vi "HardwareLoop.vi"(8 "Error In":errorcluster, 9 "Executable Configuration":T2, 10 "Data Structures":T1, 11 "Action Queues":T3) -> (0 "Error Out":errorcluster)   [LabVIEW 2012]
uses:
  ActionQueues.ctl
  UIActionQueueElement.ctl
  UIAction.ctl
  HardwareActionQueueElement.ctl
  HardwareAction.ctl
  LogActionQueueElement.ctl
  LogAction.ctl
  ExecutableConfiguration.ctl
  DataStructures.ctl
  HardwareDisplayData.ctl
  HardwareLogData.ctl
  Setup.ctl
  DUTConfiguration.ctl
  driver/Public/Controls/SMUSense.ctl
  LogConfiguration.ctl
  LogStartConfiguration.ctl
  LogStartTriggerType.ctl
  LogDigitalIOTriggerEdge.ctl
  LogRolloverConfiguration.ctl
  LogRolloverTriggerType.ctl
  LogStopConfiguration.ctl
  LogStopTriggerType.ctl
  TriggerConfiguration.ctl
  TriggerInputConfiguration.ctl
  TriggerInputType.ctl
  driver/Public/Controls/TriggerMode.ctl
  TriggerOutputConfiguration.ctl
  TriggerOutputType.ctl
  SourceConfiguration.ctl
  SourceFunction.ctl
  MeasureConfiguration.ctl
  HardwareAbortGlobalAction.ctl
  <vilib>/Utility/error.llb/DialogType.ctl
  driver/Keithley-2602.lvlib
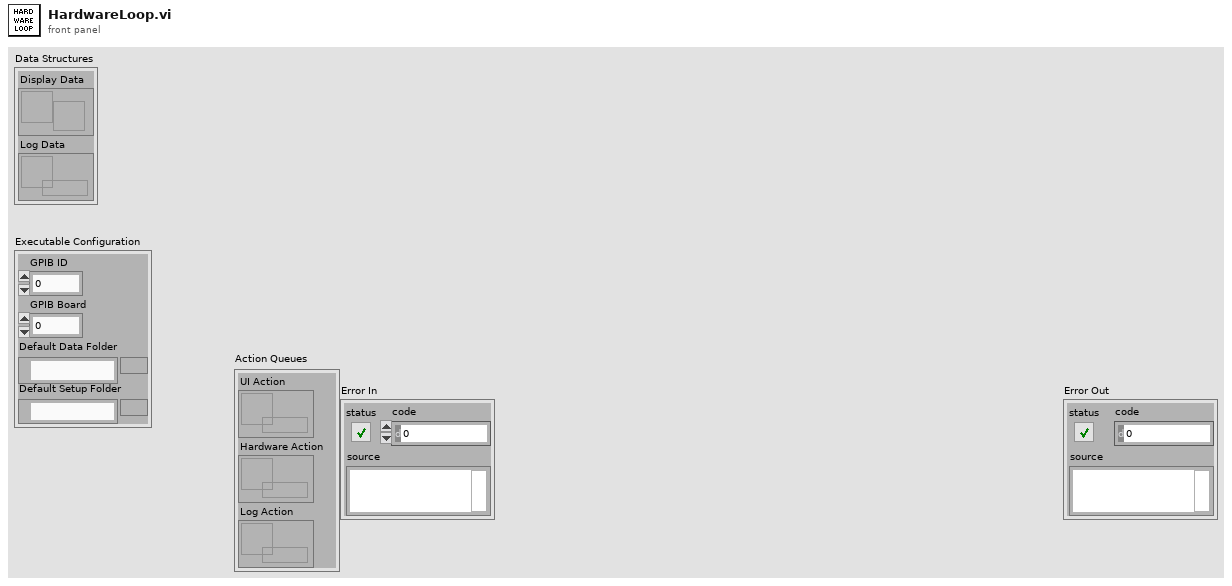
[diagram p1: front panel]
types:
  T1 = typedef "DataStructures.ctl" = cluster{"Display Data":refnum<notifier>, "Log Data":refnum<queue>}
  T2 = typedef "ExecutableConfiguration.ctl" = cluster{"GPIB ID":u8, "GPIB Board":u8, "Default Data Folder":path, "Default Setup Folder":path}
  T3 = typedef "ActionQueues.ctl" = cluster{"UI Action":refnum<queue>, "Hardware Action":refnum<queue>, "Log Action":refnum<queue>}
  T4 = typedef "Setup.ctl" = cluster{"DUT":T5, "Log":T7, "Trigger":T15, "Sources":T21[], "Measures":T23[]}
  T5 = typedef "DUTConfiguration.ctl" = cluster{"Count":u32, "Wirings":T6[], "Names":string[][]}
  T6 = typedef "Keithley-2602.lvlib/SMUSense.ctl" = enum16{"Local (2-wire)", "Remote (4-wire)", "Calibration"}
  T7 = typedef "LogConfiguration.ctl" = cluster{"Start":T8, "Rollover":T11, "Stop":T13}
  T8 = typedef "LogStartConfiguration.ctl" = cluster{"Trigger Type":T9, "Timer (sec)":dbl, "Digital IO Line":u8, "Digital IO Edge":T10}
  T9 = typedef "LogStartTriggerType.ctl" = enum16{"Immediate", "User", "Timer", "Digital IO"}
  T10 = typedef "LogDigitalIOTriggerEdge.ctl" = enum16{"Rising", "Falling"}
  T11 = typedef "LogRolloverConfiguration.ctl" = cluster{"Trigger Type":T12, "Timer (sec)":dbl, "File Size (MB)":u32, "Digital IO Line":u8, "Digital IO Edge":T10}
  T12 = typedef "LogRolloverTriggerType.ctl" = enum16{"None", "Timer", "File Size", "Digital IO"}
  T13 = typedef "LogStopConfiguration.ctl" = cluster{"Trigger Type":T14, "Timer (sec)":dbl, "File Size (MB)":u32, "Digital IO Line":u8, "Digital IO Edge":T10}
  T14 = typedef "LogStopTriggerType.ctl" = enum16{"None", "User", "Timer", "File Size", "Digital IO"}
  T15 = typedef "TriggerConfiguration.ctl" = cluster{"Input":T16, "Output":T19}
  T16 = typedef "TriggerInputConfiguration.ctl" = cluster{"Type":T17, "Timeout (ms)":u32, "Delay (ms)":u32, "Digital IO Line (1-14)":u8, "Digital IO Mode":T18}
  T17 = typedef "TriggerInputType.ctl" = enum16{"None", "Digital IO", "Bus"}
  T18 = typedef "Keithley-2602.lvlib/TriggerMode.ctl" = enum16{"Falling", "Rising", "Either", "Synchronous"}
  T19 = typedef "TriggerOutputConfiguration.ctl" = cluster{"Type":T20, "Delay (ms)":u32, "Digital IO Line (1-14)":u8, "Digital IO Mode":T18, "Digital IO Pulse Width (sec)":dbl}
  T20 = typedef "TriggerOutputType.ctl" = enum16{"None", "Digital IO", "Bus"}
  T21 = typedef "SourceConfiguration.ctl" = cluster{"Enabled?":bool, "Function":T22, "Level (V or A)":dbl, "Autorange Enabled?":bool, "High Limit (V or A)":dbl, "Low Limit (V or A)":dbl}
  T22 = typedef "SourceFunction.ctl" = enum16{"Voltage", "Current"}
  T23 = typedef "MeasureConfiguration.ctl" = cluster{"Enabled?":bool, "Count":u8, "Interval (sec)":dbl, "Voltage Auto Range Enabled?":bool, "Voltage High Limit (V or A)":dbl, "Voltage Low Limit (V or A)":dbl, "Current Auto Range Enabled?":bool, "Current High Limit (V or A)":dbl, "Current Low Limit (V or A)":dbl}
  T24 = typedef "HardwareActionQueueElement.ctl" = cluster{"Action":T25, "Data":variant}
  T25 = typedef "HardwareAction.ctl" = enum16{"Initialize", "Start", "Run", "Stop", "Error", "Shutdown"}
  T26 = typedef "UIActionQueueElement.ctl" = cluster{"Action":T27, "Data":variant}
  T27 = typedef "UIAction.ctl" = enum16{"Initialize", "Configure Trigger", "Configure Measure", "Configure Source", "Configure DUT", "Configure Log", "Configure Open", "Configure Save", "Configure Reset", "Hardware Start", "Hardware Started", "Hardware Stop", "Hardware Stopped", "Log Arm", "Log Start", "Log Started", "Log Stop", "Log Stopped", "Create Chart", "Error", "Shutdown"}
  T28 = typedef "HardwareLogData.ctl" = cluster{"Timestamp":timestamp, "Data":T29}
  T29 = typedef "HardwareDisplayData.ctl" = cluster{"DUT Names":string[][], "SMU":dbl[][], "Port":bool[]}
  T30 = typedef "HardwareAbortGlobalAction.ctl" = enum16{"Set", "Get"}
  T31 = typedef "DialogType.ctl" = u16
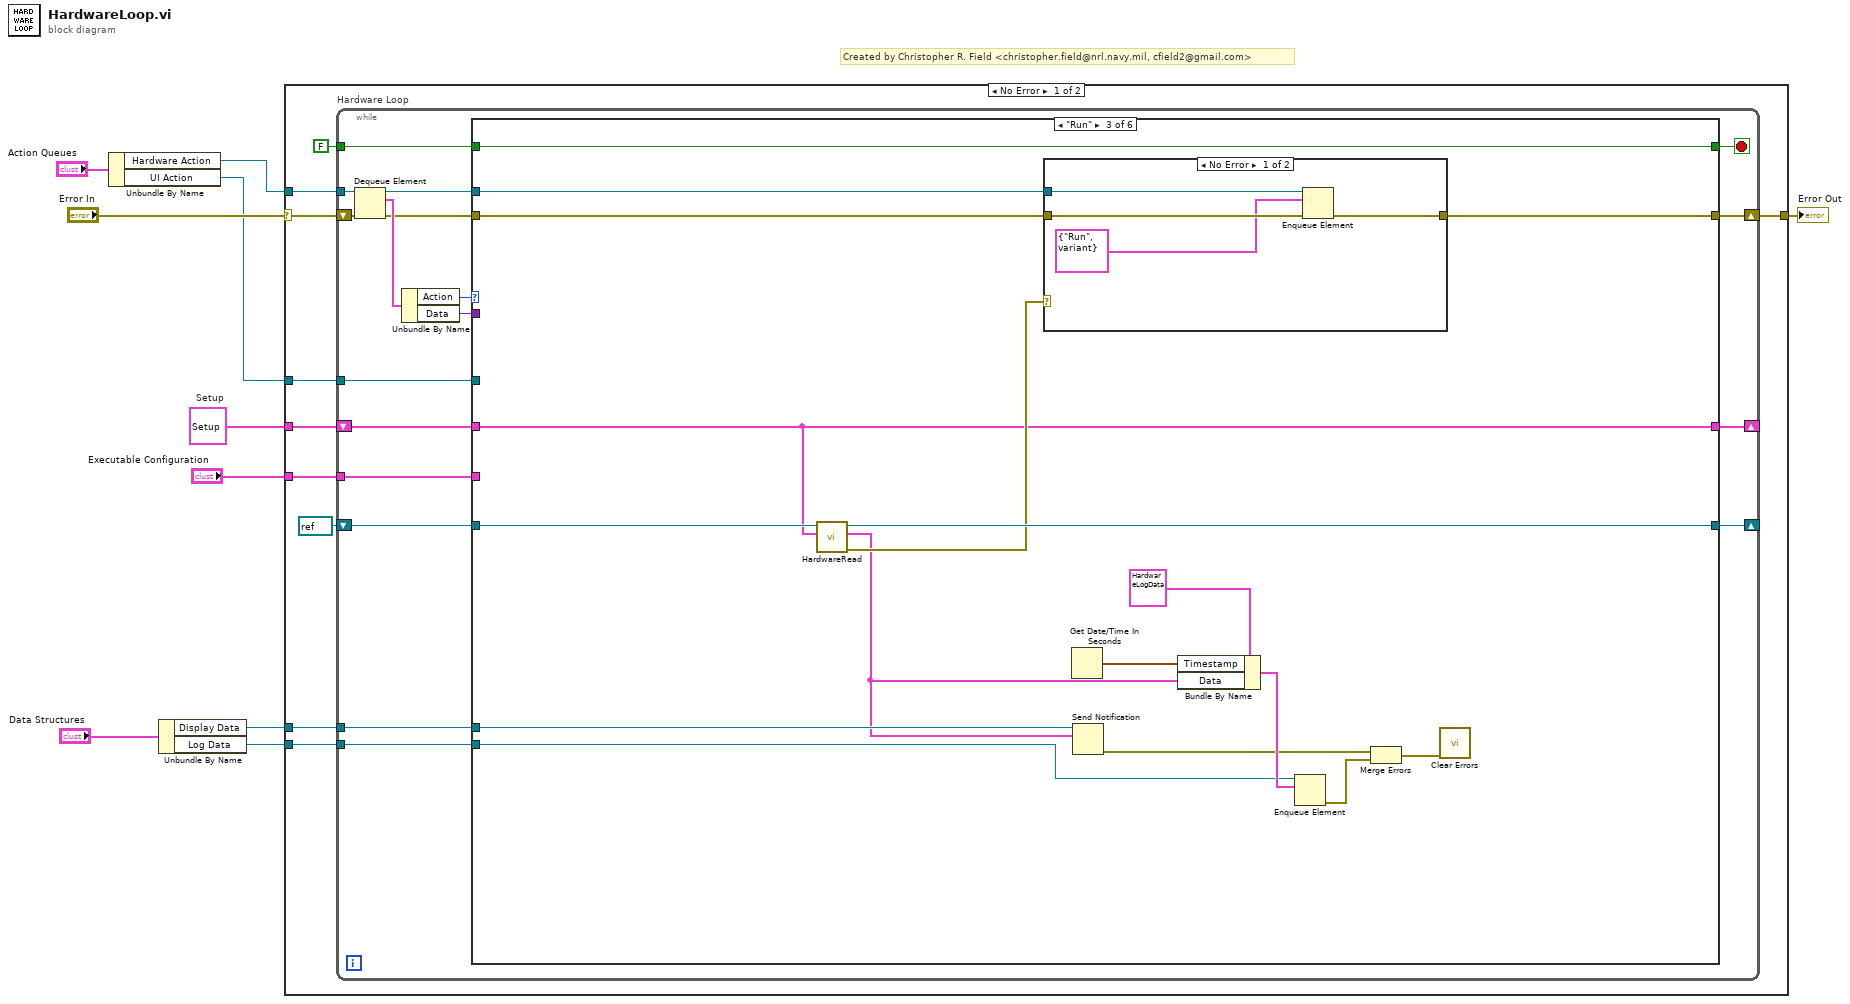
[diagram p0: block diagram]
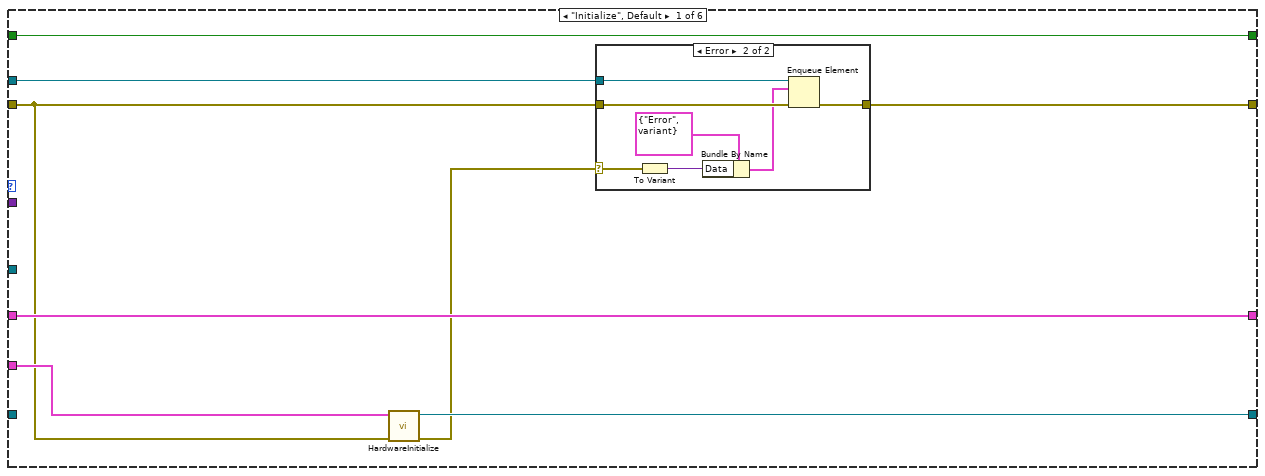
[diagram p2: hidden frame]
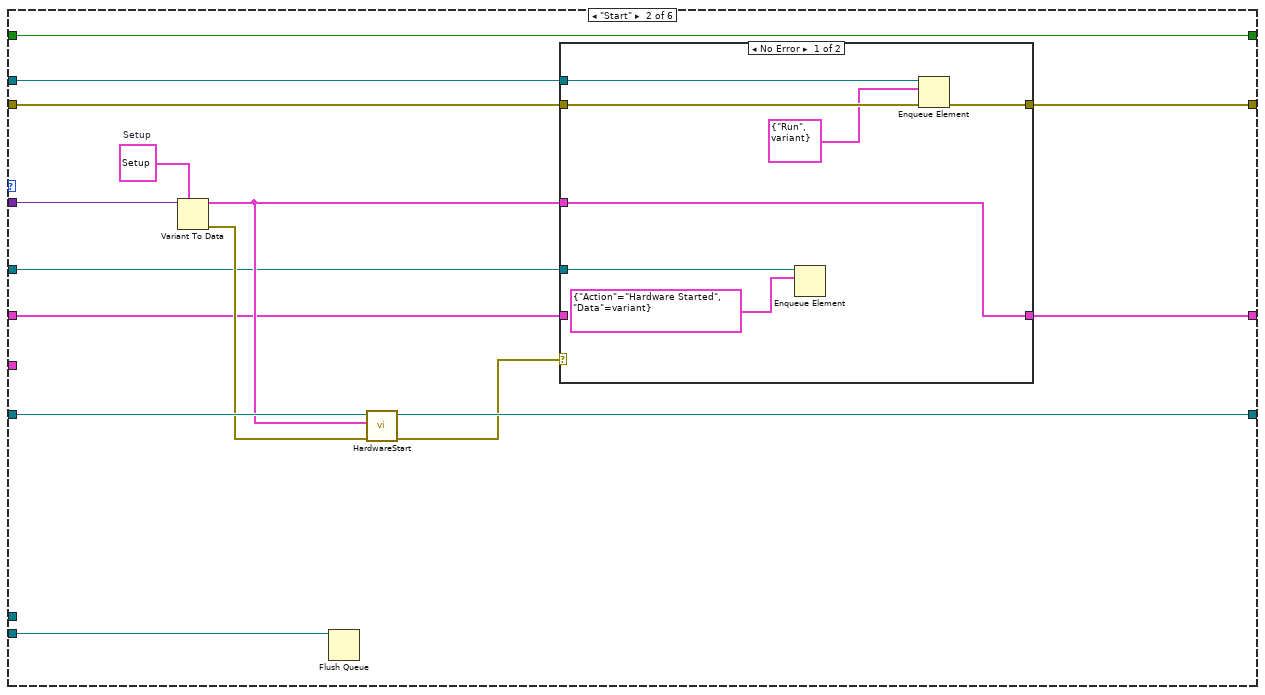
[diagram p4: hidden frame]
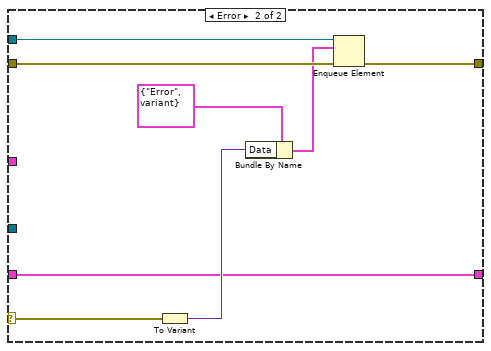
[diagram p5: hidden frame]
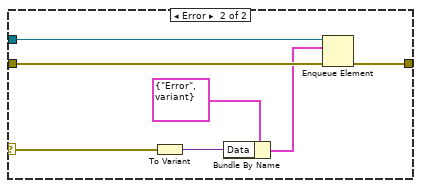
[diagram p6: hidden frame]
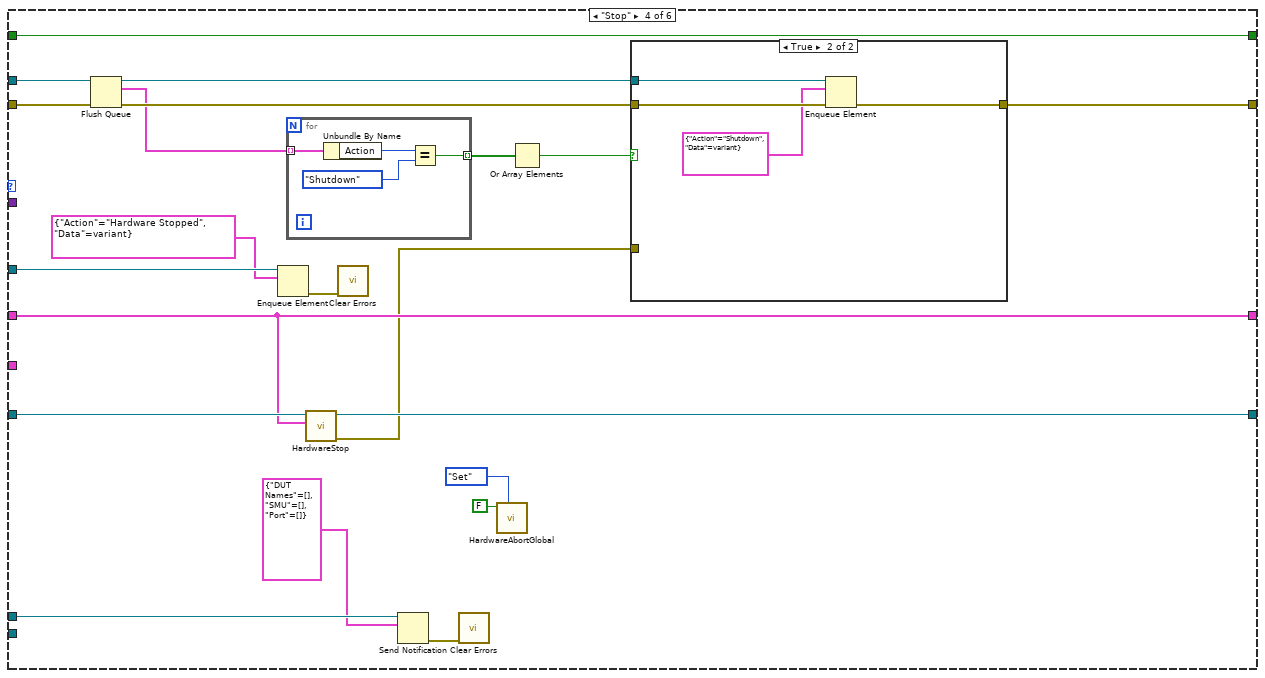
[diagram p7: hidden frame]
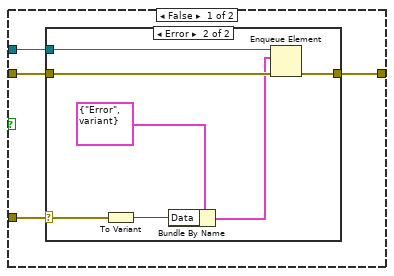
[diagram p8: hidden frame]
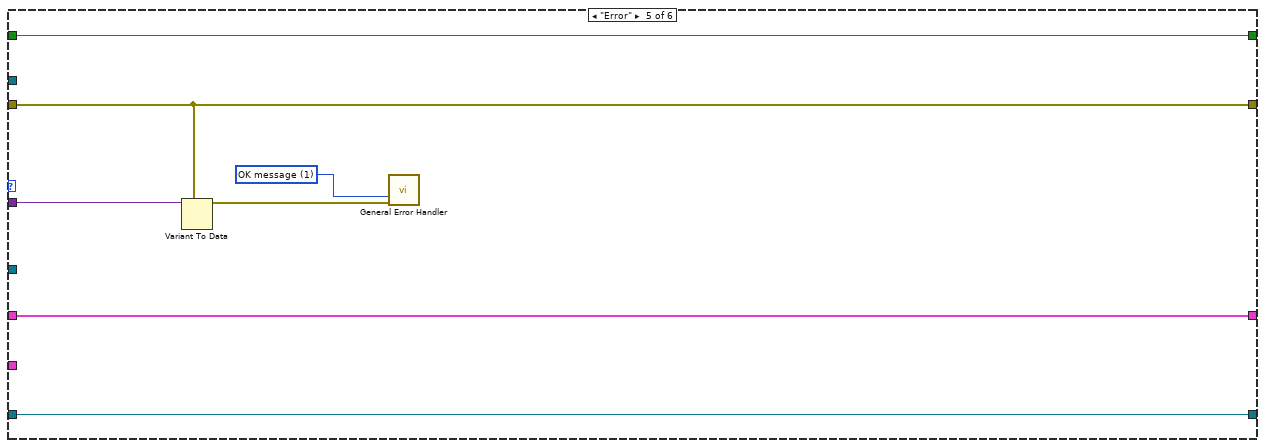
[diagram p10: hidden frame]
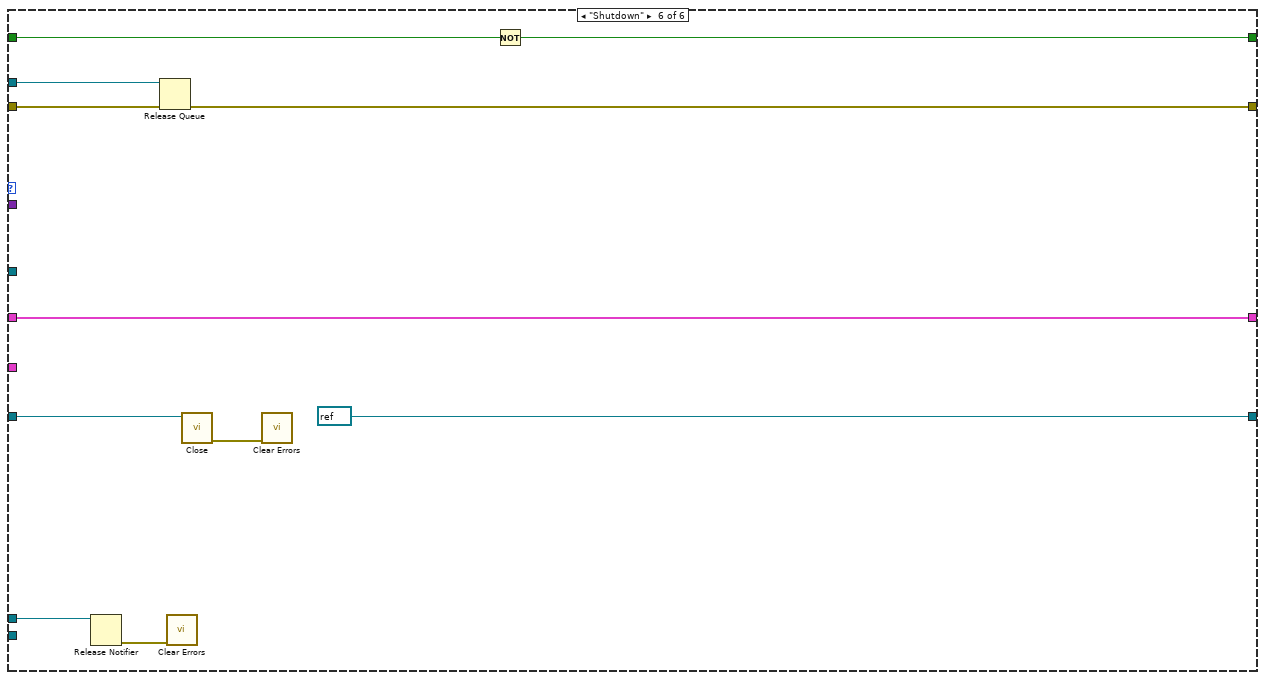
[diagram p11: hidden frame]
diagram:
  w5 = T4 {"DUT"={"Count"=0, "Wirings"=[], "Names"=[]}, "Log"={"Start"={"Trigger Type"=enum."Immediate", "Timer (sec)"=0.0, "Digital IO Line"=0, "Digital IO Edge"=enum."Rising"}, "Rollover"={"Trigger Type"=enum."None", "Timer (sec)"=0.0, "File Size (MB)"=0, "Digital IO Line"=0, "Digital IO Edge"=enum."Rising"}, "Stop"={"Trigger Type"=enum."None", "Timer (sec)"=0.0, "File Size (MB)"=0, "Digital IO Line"=0, "Digital IO Edge"=enum."Rising"}}, "Trigger"={"Input"={"Type"=enum."None", "Timeout (ms)"=0, "Delay (ms)"=0, "Digital IO Line (1-14)"=0, "Digital IO Mode"=enum."Falling"}, "Output"={"Type"=enum."None", "Delay (ms)"=0, "Digital IO Line (1-14)"=0, "Digital IO Mode"=enum."Falling", "Digital IO Pulse Width (sec)"=0.0}}, "Sources"=[], "Measures"=[]}  # Setup
  # "Created by Christopher R. Field <christopher.field@nrl.navy.mil, cfield2@gmail.com>"
  n1 = Unbundle By Name("Action Queues") -> ("Hardware Action"=w9:refnum<queue>, "UI Action"=w1:refnum<queue>)
  n2 = Unbundle By Name("Data Structures") -> ("Display Data"=w3:refnum<notifier>, "Log Data"=w2:refnum<queue>)
  n3 = case shown="No Error" "Error In" {
    selector: "Error In" -> [w19 w172]
    tunnel: w9 -> [w20 _]
    tunnel: [w17 w172] -> w7
    tunnel: "Executable Configuration" -> [w16 _]
    tunnel: w5 -> [w14 _]
    tunnel: w3 -> [w13 _]
    tunnel: w2 -> [w12 _]
    tunnel: w1 -> [w11 _]
    frame No Error {
      n4 = while "Hardware Loop" {
        tunnel: w20 -> [w38]
        shift-right: [w29] -> w17
        shift-left: w19 -> [w37]
        tunnel: FALSE -> [w31]
        tunnel: w16 -> [w28]
        shift-right: [w27] -> _
        shift-left: refnum<visa-resource-name> refnum ("Keithley 2602 Out") -> [w26]
        shift-right: [w24] -> _
        shift-left: w14 -> [w25]
        tunnel: w13 -> [w23]
        tunnel: w12 -> [w22]
        tunnel: w11 -> [w21]
        stop <- w30 stop-if-true
        n5 = Dequeue Element(queue=w38, error in (no error)=w37) -> (queue out=w32:refnum<queue>, element=w36:T24, error out=w33:errorcluster)  [unwired: 1 in, 1 out]
        n6 = Unbundle By Name(w36) -> ("Action"=w35:T25, "Data"=w34:variant)
        n7 = case shown="\"Run\"" w35 {
          tunnel: w34 -> [_ w66 _ _ w157 _]
          tunnel: w33 -> [w41 w59 w96 w118 w156 w168]
          tunnel: w32 -> [w45 w58 w97 w119 _ w169]
          tunnel: w31 -> [w46 w69 w101 w133 w160 w171]
          tunnel: [w46 w69 w101 w133 w160 w170] -> w30
          tunnel: [w44 w57 w95 w128 w156 w167] -> w29
          tunnel: w28 -> [w42 _ _ _ _ _]
          tunnel: [w40 w67 w99 w131 w159 refnum<visa-resource-name> refnum ("Keithley 2602 Out")] -> w27
          tunnel: w26 -> [_ w68 w100 w132 w159 w166]
          tunnel: w25 -> [w43 w61 w94 w130 w158 w163]
          tunnel: [w43 w60 w94 w130 w158 w163] -> w24
          tunnel: w23 -> [_ _ w93 w125 _ w162]
          tunnel: w22 -> [_ w55 w89 _ _ _]
          tunnel: w21 -> [_ w56 _ w127 _ _]
          frame "Initialize", Default {
            n8 = call "HardwareInitialize.vi"("Error In"=w41, "Executable Configuration"=w42) -> ("Error Out"=w39:errorcluster, "Keithley 2602 Out"=w40:refnum<visa-resource-name>)  [unwired: 8 in]
            n9 = case shown="Error" w39 {
              selector: w39 -> [_ w49]
              tunnel: w41 -> [w47 w53]
              tunnel: w45 -> [_ w54]
              tunnel: [w47 w52] -> w44
              frame No Error {
              }
              frame Error {
                n10 = To Variant(anything=w49) -> (Variant=w50:variant)
                n11 = Bundle By Name(cluster=T24 {"Action"=enum."Error", "Data"=variant} ("element"), "Data"=w50) -> (w48:T24)
                n12 = Enqueue Element(queue=w54, element=w48, error in (no error)=w53) -> (error out=w52:errorcluster)  [unwired: 1 in, 2 out]
              }
            }
          }
          frame "Start" {
            w65 = T4 {"DUT"={"Count"=0, "Wirings"=[], "Names"=[]}, "Log"={"Start"={"Trigger Type"=enum."Immediate", "Timer (sec)"=0.0, "Digital IO Line"=0, "Digital IO Edge"=enum."Rising"}, "Rollover"={"Trigger Type"=enum."None", "Timer (sec)"=0.0, "File Size (MB)"=0, "Digital IO Line"=0, "Digital IO Edge"=enum."Rising"}, "Stop"={"Trigger Type"=enum."None", "Timer (sec)"=0.0, "File Size (MB)"=0, "Digital IO Line"=0, "Digital IO Edge"=enum."Rising"}}, "Trigger"={"Input"={"Type"=enum."None", "Timeout (ms)"=0, "Delay (ms)"=0, "Digital IO Line (1-14)"=0, "Digital IO Mode"=enum."Falling"}, "Output"={"Type"=enum."None", "Delay (ms)"=0, "Digital IO Line (1-14)"=0, "Digital IO Mode"=enum."Falling", "Digital IO Pulse Width (sec)"=0.0}}, "Sources"=[], "Measures"=[]}  # Setup
            n13 = Variant To Data(type=w65, Variant=w66) -> (data=w63:T4, error out=w64:errorcluster)  [unwired: 1 in]
            n14 = Flush Queue(queue=w55) -> ()  [unwired: 1 in, 3 out]
            n15 = call "HardwareStart.vi"("Error In"=w64, "Hardware Configuration"=w63, "Keithley 2602 In"=w68) -> ("Error Out"=w62:errorcluster, "Keithley 2602 Out"=w67:refnum<visa-resource-name>)  [unwired: 7 in]
            n16 = case shown="No Error" w62 {
              selector: w62 -> [_ w79]
              tunnel: w63 -> [w76 _]
              tunnel: [w76 w77] -> w60
              tunnel: w61 -> [_ w77]
              tunnel: w59 -> [w74 w83]
              tunnel: w58 -> [w75 w84]
              tunnel: [w73 w82] -> w57
              tunnel: w56 -> [w71 _]
              frame No Error {
                n17 = Enqueue Element(queue=w71, element=T26 {"Action"=enum."Hardware Started", "Data"=variant}) -> ()  [unwired: 2 in, 3 out]
                n18 = Enqueue Element(queue=w75, element=T24 {"Action"=enum."Run", "Data"=variant}, error in (no error)=w74) -> (error out=w73:errorcluster)  [unwired: 1 in, 2 out]
              }
              frame Error {
                n19 = To Variant(anything=w79) -> (Variant=w80:variant)
                n20 = Bundle By Name(cluster=T24 {"Action"=enum."Error", "Data"=variant} ("element"), "Data"=w80) -> (w78:T24)
                n21 = Enqueue Element(queue=w84, element=w78, error in (no error)=w83) -> (error out=w82:errorcluster)  [unwired: 1 in, 2 out]
              }
            }
          }
          frame "Run" {
            n22 = call "HardwareRead.vi"("Hardware Configuration"=w94, "Keithley 2602 In"=w100) -> ("Error Out"=w98:errorcluster, "Hardware Display Data"=w88:T29, "Keithley 2602 Out"=w99:refnum<visa-resource-name>)  [unwired: 7 in]
            n23 = case shown="No Error" w98 {
              selector: w98 -> [_ w107]
              tunnel: w97 -> [w105 w112]
              tunnel: w96 -> [w104 w111]
              tunnel: [w103 w110] -> w95
              frame No Error {
                n24 = Enqueue Element(queue=w105, element=T24 {"Action"=enum."Run", "Data"=variant}, error in (no error)=w104) -> (error out=w103:errorcluster)  [unwired: 1 in, 2 out]
              }
              frame Error {
                n25 = To Variant(anything=w107) -> (Variant=w108:variant)
                n26 = Bundle By Name(cluster=T24 {"Action"=enum."Error", "Data"=variant} ("element"), "Data"=w108) -> (w106:T24)
                n27 = Enqueue Element(queue=w112, element=w106, error in (no error)=w111) -> (error out=w110:errorcluster)  [unwired: 1 in, 2 out]
              }
            }
            n28 = Get Date/Time In Seconds() -> (seconds since 1Jan1904=w91:timestamp)
            n29 = Send Notification(notification=w88, notifier=w93) -> (error out=w87:errorcluster)  [unwired: 1 in, 1 out]
            n30 = Bundle By Name(cluster=T28 {"Timestamp"=timestamp(0 s since 1904-01-01), "Data"={"DUT Names"=[], "SMU"=[], "Port"=[]}} ("Hardware Log Data"), "Timestamp"=w91, "Data"=w88) -> (w90:T28)
            n31 = Enqueue Element(queue=w89, element=w90) -> (error out=w86:errorcluster)  [unwired: 2 in, 2 out]
            n32 = Merge Errors(w87, w86) -> (w85:errorcluster)
            n33 = call <vilib>:"Clear Errors.vi"("error in (no error)"=w85) -> ()  [unwired: 6 in, 1 out]
          }
          frame "Stop" {
            n34 = Flush Queue(queue=w119, error in (no error)=w118) -> (queue out=w116:refnum<queue>, remaining elements=w115:T24[], error out=w117:errorcluster)
            n35 = Enqueue Element(queue=w127, element=T26 {"Action"=enum."Hardware Stopped", "Data"=variant}) -> (error out=w123:errorcluster)  [unwired: 2 in, 2 out]
            n36 = for {
              tunnel: w115 -> [w153] mode=indexing
              tunnel: [w150] -> w114 mode=indexing
              n37 = Unbundle By Name(w153) -> ("Action"=w152:T25)
              n38 = Equal?(x=w152, y=HardwareAction."Shutdown") -> (x = y?=w150:bool)
            }
            n39 = call "HardwareStop.vi"("Hardware Configuration"=w130, "Keithley 2602 In"=w132) -> ("Error Out"=w129:errorcluster, "Keithley 2602 Out"=w131:refnum<visa-resource-name>)  [unwired: 8 in]
            n40 = call <vilib>:"Clear Errors.vi"("error in (no error)"=w123) -> ()  [unwired: 6 in, 1 out]
            n41 = Send Notification(notification=T29 {"DUT Names"=[], "SMU"=[], "Port"=[]}, notifier=w125) -> (error out=w122:errorcluster)  [unwired: 1 in, 1 out]
            n42 = call <vilib>:"Clear Errors.vi"("error in (no error)"=w122) -> ()  [unwired: 6 in, 1 out]
            n43 = call "HardwareAbortGlobal.vi"("Action"=HardwareAbortGlobalAction."Set", "Set Value"=FALSE) -> ()  [unwired: 9 in, 1 out]
            n44 = Or Array Elements(Boolean array=w114) -> (logical OR=w113:bool)
            n45 = case shown="True" w113 {
              tunnel: w129 -> [w137 _]
              tunnel: [w136 w147] -> w128
              tunnel: w117 -> [w135 w148]
              tunnel: w116 -> [w134 w149]
              frame False {
                n46 = case shown="Error" w137 {
                  selector: w137 -> [_ w141]
                  tunnel: w135 -> [w138 w144]
                  tunnel: w134 -> [_ w145]
                  tunnel: [w138 w139] -> w136
                  frame No Error {
                  }
                  frame Error {
                    n47 = To Variant(anything=w141) -> (Variant=w142:variant)
                    n48 = Bundle By Name(cluster=T24 {"Action"=enum."Error", "Data"=variant} ("element"), "Data"=w142) -> (w140:T24)
                    n49 = Enqueue Element(queue=w145, element=w140, error in (no error)=w144) -> (error out=w139:errorcluster)  [unwired: 1 in, 2 out]
                  }
                }
              }
              frame True {
                n50 = Enqueue Element(queue=w149, element=T24 {"Action"=enum."Shutdown", "Data"=variant}, error in (no error)=w148) -> (error out=w147:errorcluster)  [unwired: 1 in, 2 out]
              }
            }
          }
          frame "Error" {
            w154 = T31 1 items=["no dialog", "OK message", "continue or stop message", "OK message + warnings", "continue/stop + warnings"] ("type of dialog (OK msg:1)")
            n51 = Variant To Data(type=w156, Variant=w157) -> (data=w155:errorcluster)  [unwired: 1 in, 1 out]
            n52 = call <vilib>:"General Error Handler.vi"("type of dialog (OK msg:1)"=w154, "error in (no error)"=w155) -> ()  [unwired: 9 in, 5 out]
          }
          frame "Shutdown" {
            n53 = Release Notifier(notifier=w162) -> (error out=w161:errorcluster)  [unwired: 2 in, 2 out]
            n54 = Release Queue(queue=w169, error in (no error)=w168) -> (error out=w167:errorcluster)  [unwired: 1 in, 2 out]
            n55 = call <vilib>:"Clear Errors.vi"("error in (no error)"=w161) -> ()  [unwired: 6 in, 1 out]
            n56 = call "Close.vi"("Keithley 2602 In"=w166) -> ("Error Out"=w165:errorcluster)  [unwired: 10 in]
            n57 = call <vilib>:"Clear Errors.vi"("error in (no error)"=w165) -> ()  [unwired: 6 in, 1 out]
            n58 = Not(x=w171) -> (.not. x?=w170:bool)
          }
        }
      }
    }
    frame Error {
    }
  }
  "Error Out" <- w7
